vi "Create Interface.vi"(7 "App Inst":refnum<vi>, 8 "error in (no error)":errorcluster, 9 "Actor Name":string, 11 "Library in":refnum<vi>) -> (0 "error out":errorcluster, 3 "Library out":refnum<vi>)   [LabVIEW 2020, in "Add Actor Interface.lvlib"]
uses:
  Add Actor Interface.lvlib
  <vilib>/Utility/EditLVLibs/Edit LVLibs.lvlib
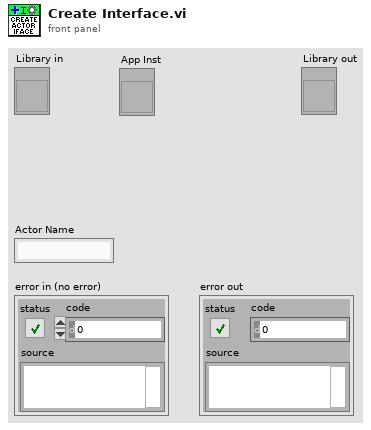
[diagram p1: front panel]
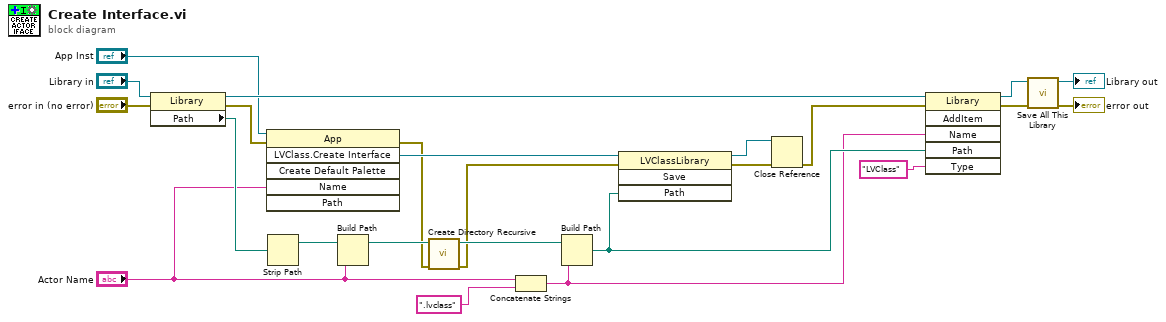
[diagram p0: block diagram]
diagram:
  n1 = property class="Library"(reference="Library in", error in="error in (no error)") -> (reference out=w23:refnum<vi>, error out=w17:errorcluster, "Path"=w21:path)
  n2 = invoke class="App" method="LVClass.Create Interface"(reference="App Inst", error in=w17, "Name"="Actor Name") -> (error out=w7:errorcluster, "LVClass.Create Interface"=w16:refnum<vi>)  [unwired: 3 in, 4 out]
  n3 = Strip Path(path=w21) -> (stripped path=w12:path)  [unwired: 1 out]
  n4 = Build Path(base path=w12, name or relative path="Actor Name") -> (appended path=w9:path)
  n5 = call <vilib>:"Create Directory Recursive.vi"("error in (no error)"=w7, "directory"=w9) -> ("error out"=w6:errorcluster, "directory copy"=w8:path)  [unwired: 3 in, 1 out]
  n6 = Concatenate Strings("Actor Name", ".lvclass" ("string")) -> (w10:string)
  n7 = Build Path(base path=w8, name or relative path=w10) -> (appended path=w19:path)
  n8 = invoke class="LVClassLibrary" method="Save"(reference=w16, error in=w6, "Path"=w19) -> (reference out=w15:refnum<vi>, error out=w14:errorcluster)  [unwired: 1 in, 2 out]
  n9 = Close Reference(reference=w15, error in (no error)=w14) -> (error out=w13:errorcluster)
  n10 = invoke class="Library" method="AddItem"(reference=w23, error in=w13, "Name"=w10, "Path"=w19, "Type"="LVClass") -> (reference out=w2:refnum<vi>, error out=w4:errorcluster)  [unwired: 1 in, 4 out]
  n11 = call <vilib>:"Save All This Library.vi"("error in (no error)"=w4, "Library in"=w2) -> ("error out"=→"error out":errorcluster, "Library out"=→"Library out":refnum<vi>)  [unwired: 8 in]
